vi "Calibrated Distance to Hood Angle.vi"(8 "error in (no error)":errorcluster, 10 "Calibration (DISTANCE MUST BE MONOTONIC)":cluster{"Distance":dbl, "Hood Angle":dbl}[](array[cluster]), 11 "Distance":dbl) -> (0 "error out":errorcluster, 3 "Hood Angle":dbl)   [LabVIEW 2019]
uses:
  <vilib>/gmath/NI_Gmath.lvlib
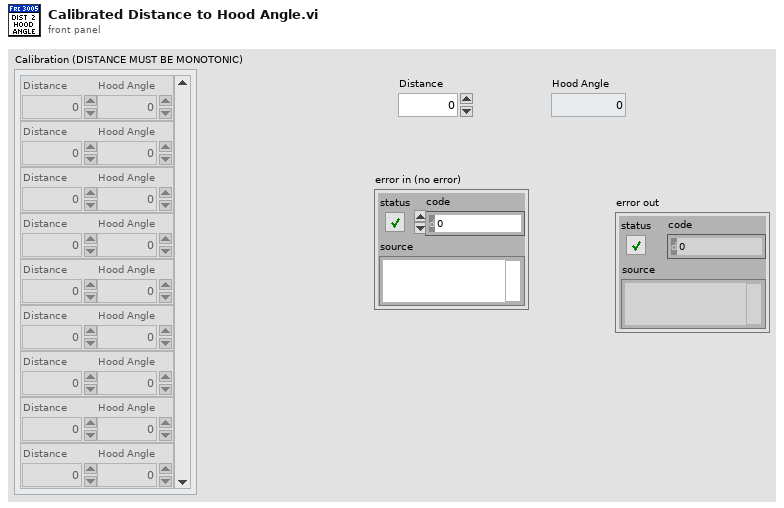
[diagram p1: front panel]
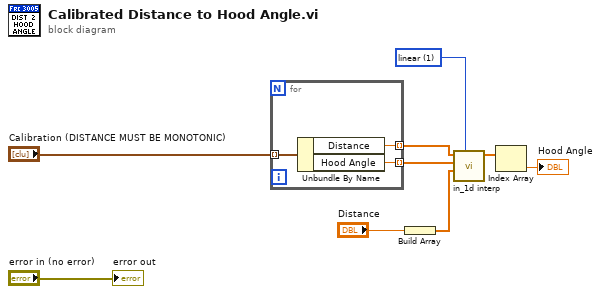
[diagram p0: block diagram]
diagram:
  w9 = 1 items=["nearest", "linear", "spline", "cubic Hermite", "Lagrange"] ("method")
  n1 = for {
    tunnel: "Calibration (DISTANCE MUST BE MONOTONIC)" -> [w12] mode=indexing
    tunnel: [w11] -> w2 mode=indexing
    tunnel: [w10] -> w1 mode=indexing
    n2 = Unbundle By Name(w12) -> ("Distance"=w11:dbl, "Hood Angle"=w10:dbl)
  }
  n3 = Build Array("Distance") -> (w7:dbl[])
  n4 = call <vilib>:"in_1d interp.vi"("method"=w9, "xi"=w7, "Y"=w1, "X"=w2) -> ("yi"=w6:dbl[])  [unwired: 6 in, 1 out]
  n5 = Index Array(array=w6) -> (element=→"Hood Angle":dbl)  [unwired: 1 in]
  "error out" <- "error in (no error)"
